vi "Dynamic Launch CaseSelect.vi"(8 "error in (no error)":errorcluster, 10 "Active VI Sel. List[]":refnum<vi>[](array[refnum])) -> (0 "error out":errorcluster)   [LabVIEW 2020]
uses:
  JKI State Machine API/source/JKI SM/JKI SM.lvclass
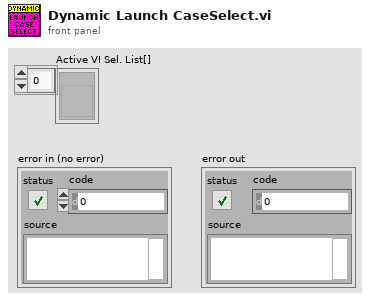
[diagram p1: front panel]
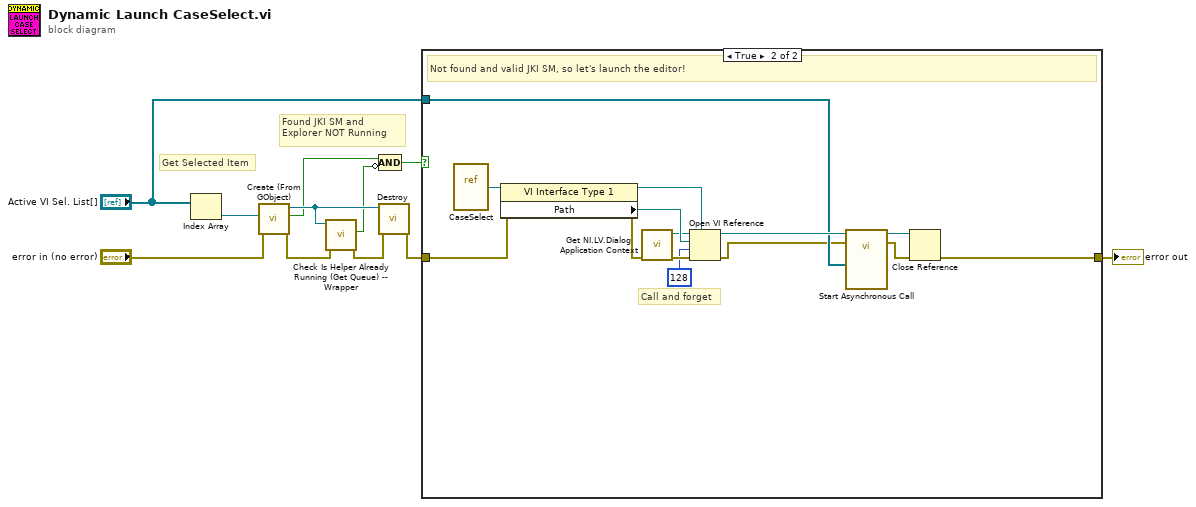
[diagram p0: block diagram]
diagram:
  # "Found JKI SM and Explorer NOT Running"
  # "Get Selected Item"
  n1 = Index Array(array="Active VI Sel. List[]") -> (element=w9:refnum<vi>)  [unwired: 1 in]
  n2 = call "Create (From GObject).vi"("error in (no error)"="error in (no error)", "GObject"=w9) -> ("error out"=w7:errorcluster, "Found JKI SMs?"=w3:bool, "JKI SM out"=w4:refnum<class "JKI SM.lvclass">)  [unwired: 6 in, 1 out]
  n3 = call "Check Is Helper Already Running (Get Queue) -- Wrapper.vi"("error in (no error)"=w7, "JKI SM in"=w4) -> ("error out"=w6:errorcluster, "is Running?"=w2:bool)  [unwired: 8 in]
  n4 = Compound Arithmetic op=AND(w3, invert w2) -> (w1:bool)
  n5 = call "Destroy.vi"("error in (no error)"=w6, "JKI SM in"=w4) -> ("error out"=w5:errorcluster)  [unwired: 9 in]
  n6 = case shown="True" w1 {
    tunnel: w5 -> [w12 w20]
    tunnel: "Active VI Sel. List[]" -> [_ w16]
    tunnel: [w12 w14] -> w10
    frame False {
      # "Don't launch another copy"
    }
    frame True {
      # "Call and forget"
      # "Not found and valid JKI SM, so let's launch the editor!"
      n7 = vi-ref "CaseSelect.vi"() -> (w26:refnum<vi>)
      n8 = property class="VI Interface Type 1"(reference=w26, error in=w20) -> (reference out=w24:refnum<vi>, error out=w19:errorcluster, "Path"=w25:path)
      n9 = call "Get NI.LV.Dialog Application Context.vi"("error in (no error)"=w19) -> ("error out"=w18:errorcluster, "Application out"=w17:refnum<vi>)  [unwired: 9 in]
      n10 = Open VI Reference(type specifier VI Refnum (for type only)=w24, application reference (local)=w17, vi path=w25, options=128, error in (no error)=w18) -> (vi reference=w23:refnum<vi>, error out=w13:errorcluster)  [unwired: 1 in]
      n11 = call-by-ref "Start Asynchronous Call"(reference=w23, error in=w13, "SelList[]"=w16) -> (reference out=w22:refnum<vi>, error out=w21:errorcluster)  [unwired: 11 in]
      n12 = Close Reference(reference=w22, error in (no error)=w21) -> (error out=w14:errorcluster)
    }
  }
  "error out" <- w10
